vi "Add Instruments.vi"(8 "Error In":errorcluster, 10 "Source":string, 11 "reference in":refnum<class "Instrument Manager.lvclass">) -> (0 "Error Out":errorcluster, 3 "reference out":refnum<class "Instrument Manager.lvclass">)   [LabVIEW 2024, in "Instrument Manager.lvclass"]
uses:
  Instrument Manager.lvclass
  Instrument Manager.lvclass/Instrument Manager.ctl
  Config from JSON/Config from JSON.lvclass
  Config from XML/Config from XML.lvclass
  Interfaces/IConfiguration/IConfiguration.lvclass
  130842e4-efc9-4244-b670-89843b52b0e0.vi
  D:/git/HAL/Source/Config from XML/Config from XML.lvclass
  D:/git/HAL/Source/Interfaces/IConfiguration/IConfiguration.lvclass
  D:/git/HAL/Source/Config from JSON/Config from JSON.lvclass
panel:
  out "Array of Data":string[](array[string])
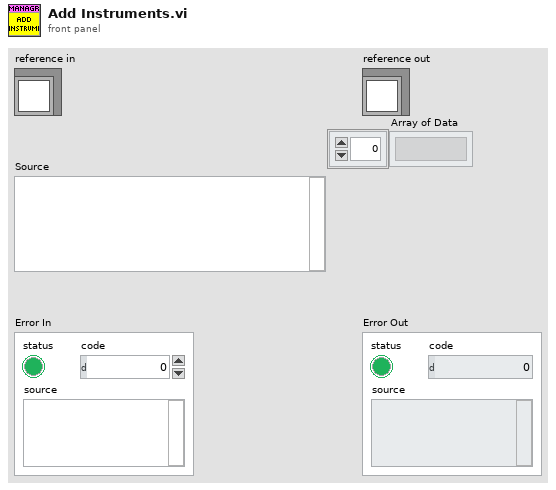
[diagram p1: front panel]
types:
  T1 = typedef "Instrument Manager.lvclass/ObjectAttributes.ctl" = cluster{"Instruments":map{string, refnum<class "IInstrument.lvclass">}}
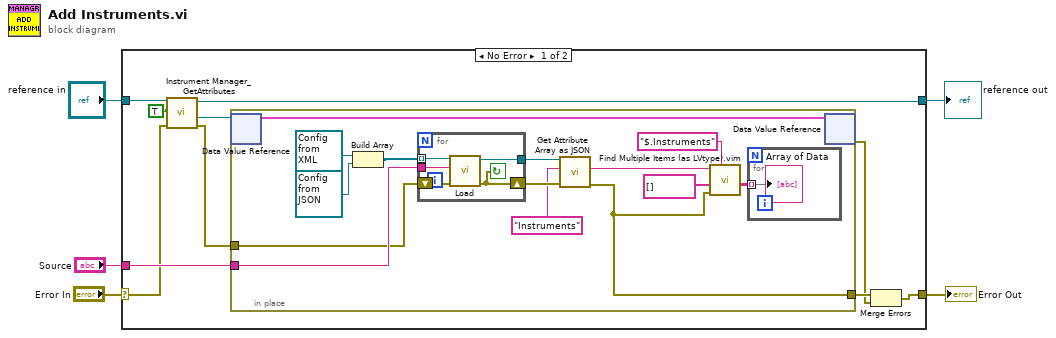
[diagram p0: block diagram]
diagram:
  n1 = case shown="No Error" "Error In" {
    selector: "Error In" -> [w12 w37]
    tunnel: [w7 w37] -> w4
    tunnel: "reference in" -> [w14 w36]
    tunnel: [w8 w36] -> w2
    tunnel: "Source" -> [w15 _]
    frame No Error {
      n2 = call "Instrument Manager_GetAttributes.vi"("Error In"=w12, "OnlyGetDvrReference(False)"=TRUE, "reference in"=w14) -> ("Error Out"=w11:errorcluster, "DataRef"=w9:refnum<data-value>, "reference out"=w8:refnum<class "Instrument Manager.lvclass">)  [unwired: 5 in, 1 out]
      n3 = in-place {
        in-place-border: w15 -> [w26]
        in-place-border: w11 -> [w25]
        in-place-border: [w19] -> w10
        n4 = in-place-dvr #1(w9) -> (w17:T1)  [unwired: 1 out]
        n5 = Build Array(refnum<class "Config from XML.lvclass"> refnum ("Config from XML.lvclass"), refnum<class "Config from JSON.lvclass"> refnum ("Config from JSON.lvclass")) -> (w27:refnum<class "IConfiguration.lvclass">[])
        n6 = for {
          tunnel: w27 -> [w32] mode=indexing
          tunnel: w26 -> [w35]
          shift-right: [w31] -> w23
          shift-left: w25 -> [w34]
          tunnel: [w33] -> w24
          stop <- w31 continue-if-true
          n7 = call-dynamic "Load.vi"("error in"=w34, "Source"=w35, "IConfiguration in"=w32) -> ("error out"=w31:errorcluster, "IConfiguration out"=w33:refnum<class "IConfiguration.lvclass">)  [unwired: 7 in]
        }
        n8 = call-dynamic "Get Attribute Array as JSON.vi"("error in"=w23, "Attribute"="Instruments", "IConfiguration in"=w24) -> ("error out"=w19:errorcluster, "<JSON>"=w21:string)  [unwired: 6 in, 1 out]
        n9 = call "Find Multiple Items (as LVtype).vim"("$Path or Item Name"="$.Instruments", "error in (no error)"=w19, "Data Type and Default Value"=string[] [], "JSON"=w21) -> ("Array of Data"=w18:string[][])  [unwired: 4 in, 3 out]
        n10 = for {
          tunnel: w18 -> [w30] mode=indexing
          "Array of Data" <- w30
        }
        n11 = in-place-dvr #1(w17) -> (w6:errorcluster)  [unwired: 1 out]
      }
      n12 = Merge Errors(w10, w6) -> (w7:errorcluster)
    }
    frame Error {
    }
  }
  "Error Out" <- w4
  "reference out" <- w2
